vi "SetParentCall.vi"(8 "error in (no error)":errorcluster, 10 "Parent Call":T1, 11 "SMO in":refnum<class "SMO.lvclass">) -> (0 "error out":errorcluster, 3 "SMO out":refnum<class "SMO.lvclass">)   [LabVIEW 2021, in "smo.lvlib" / "SMO.lvclass"]
uses:
  SMO.lvclass
  Typedefs/Parent Call--Enum.ctl
  SMO.lvclass/SMO.ctl
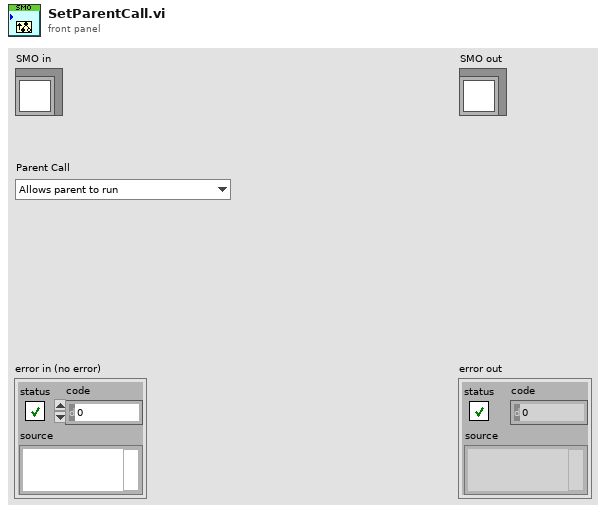
[diagram p1: front panel]
types:
  T1 = typedef "smo.lvlib/SMO.lvclass/Parent Call--Enum.ctl" = enum16{"Allows parent to run", "Does not request parent to run"}
  T2 = typedef "smo.lvlib/SMO.lvclass/PrivateData--Ref.ctl" = refnum<data-value>
  T3 = typedef "smo.lvlib/SMO.lvclass/PrivateData--Cluster.ctl" = cluster{"Parent Call":T1, "Registered Processes":T4[], "Sync Notifier":refnum<notifier>, "Process Error Notifier":refnum<notifier>, "Protected Events":T5, "Public Events":T6, "SMO State":T7, "[Attributes]":variant, "Launcher Close":refnum<notifier>, "Caller Watchdog":refnum<queue>, "Accessibility":T8, "NbStaticDependencies":u32}
  T4 = typedef "smo.lvlib/SMO.lvclass/RegisteredProcessData--Cluster.ctl" = cluster{"Name":string, "Static VI Ref":refnum<vi>, "Running":bool, "NotifierRef":u32}
  T5 = typedef "smo.lvlib/SMO.lvclass/Protected Events.ctl" = cluster{"StopProcesses":refnum<user-event>, "AbortProcesses":refnum<user-event>, "Config Changed":refnum<user-event>, "Dependency":refnum<user-event>}
  T6 = typedef "smo.lvlib/SMO.lvclass/Public Events.ctl" = cluster{"Error":refnum<user-event>, "State":refnum<user-event>, "Reserve State":refnum<user-event>}
  T7 = typedef "smo.lvlib/SMO.lvclass/SMOState --Enum.ctl" = enum16{"unknown", "Created", "Started", "Stopped"}
  T8 = typedef "smo.lvlib/SMO.lvclass/Accessibility--Cluster.ctl" = cluster{"Lock Key":string, "Reserve State":T9}
  T9 = typedef "smo.lvlib/SMO.lvclass/Reserve State--Enum.ctl" = enum16{"Unreserved", "Reserved", "Self-locked"}
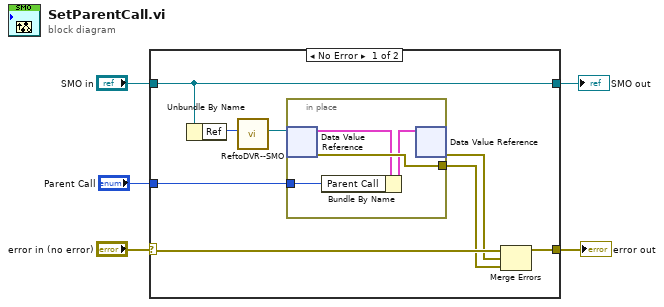
[diagram p0: block diagram]
diagram:
  n1 = case shown="No Error" "error in (no error)" {
    selector: "error in (no error)" -> [w13 w19]
    tunnel: [w12 w19] -> w2
    tunnel: [w6 w18] -> w1
    tunnel: "SMO in" -> [w6 w18]
    tunnel: "Parent Call" -> [w9 _]
    frame No Error {
      n2 = Unbundle By Name(w6) -> ("Ref"=w8:u32)
      n3 = call "ReftoDVR--SMO.vi"("Ref"=w8) -> ("Ref"=w7:T2)  [unwired: 10 in]
      n4 = in-place {
        in-place-border: [w17] -> w10
        in-place-border: w9 -> [w14]
        n5 = in-place-dvr #1(w7) -> (w16:T3, w17:errorcluster)
        n6 = Bundle By Name(cluster=w16, "Parent Call"=w14) -> (w15:T3)
        n7 = in-place-dvr #1(w15) -> (w11:errorcluster)  [unwired: 1 out]
      }
      n8 = Merge Errors(w13, w11, w10) -> (w12:errorcluster)
    }
    frame Error {
    }
  }
  "error out" <- w2
  "SMO out" <- w1
